vi "Setup Model.vi"(8 "error in (no error)":errorcluster, 9 "User Events in":refnum<class "User Events.lvclass">, 11 "Boot Loader in":refnum<class "Boot Loader.lvclass">) -> (0 "error out":errorcluster, 1 "User Events out":refnum<class "User Events.lvclass">, 2 "Model out":refnum<class "Model.lvclass">, 3 "Boot Loader out":refnum<class "Boot Loader.lvclass">)   [LabVIEW 2016, in "Boot Loader.lvclass"]
uses:
  Boot Loader.lvclass
  Model/Model.lvclass
  User Events/User Events.lvclass
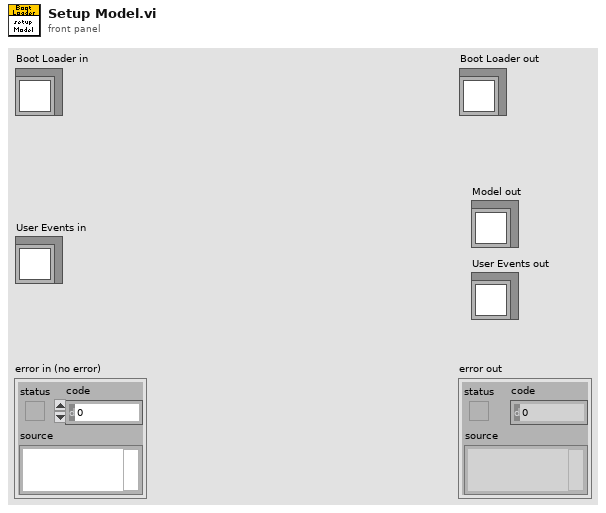
[diagram p1: front panel]
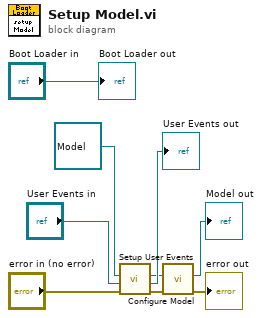
[diagram p0: block diagram]
diagram:
  n1 = call "Setup User Events.vi"("error in (no error)"="error in (no error)", "User Events in"="User Events in", "Model in"=refnum<class "Model.lvclass"> refnum) -> ("error out"=w1:errorcluster, "User Events out"=→"User Events out":refnum<class "User Events.lvclass">, "Model out"=w4:refnum<class "Model.lvclass">)  [unwired: 5 in, 1 out]
  n2 = call "Configure Model.vi"("error in (no error)"=w1, "Model in"=w4) -> ("error out"=→"error out":errorcluster, "Model out"=→"Model out":refnum<class "Model.lvclass">)  [unwired: 7 in, 1 out]
  "Boot Loader out" <- "Boot Loader in"
